vi "ROI_def.vi"(8 "pic path":path, 11 "read image      take pic":bool) -> (0 "Global Rectangle":i32[](array[numeric]), 2 "Image Out 2":T1, 3 "output cluster":cluster{i32, i32, i32, i32})   [LabVIEW 2017]
uses:
  <vilib>/vision/Image Controls.llb/IMAQ Image.ctl
panel:
  in  "Stop (F)":bool
  out "Image Out":T1(plugin-control)
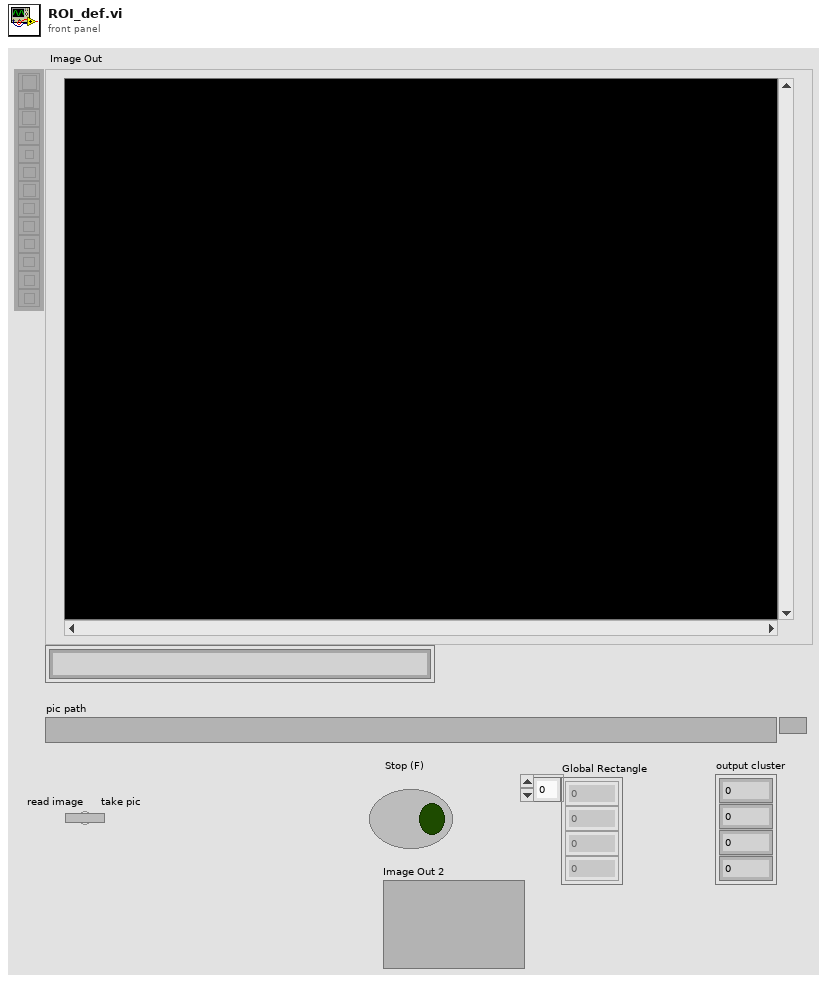
[diagram p1: front panel]
types:
  T1 = typedef "IMAQ Image.ctl" = refnum<image>
  T2 = typedef "ROI Descriptor" = cluster{"Global Rectangle":i32[], "Contours":cluster{"ID":enum32{"External", "Internal"}, "Type":u32, "Coordinates":i32[]}[]}
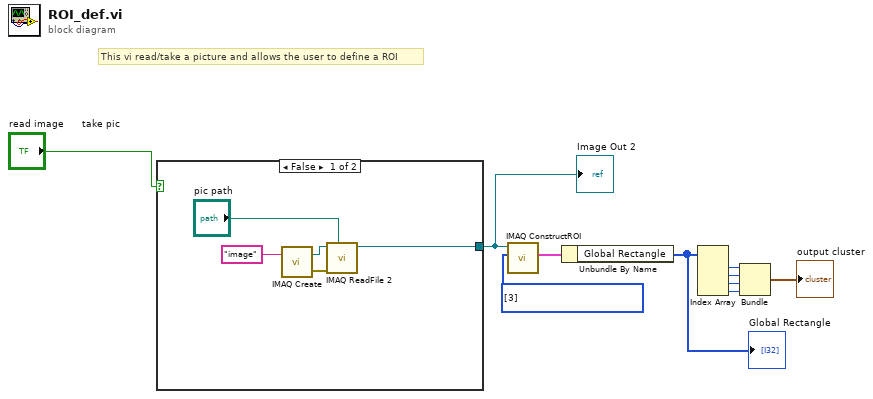
[diagram p0: block diagram]
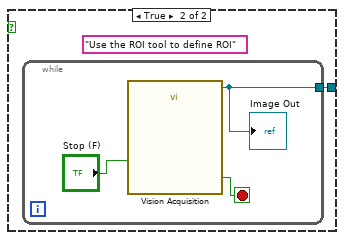
[diagram p2: hidden frame]
diagram:
  w4 = u32[] [3] items=["No Selection", "Point", "Line", "Rectangle", "Oval", "Polygon", "Freehand Region", "Annulus", "Zoom", "Pan", "Broken Line", "Freehand Line", "Rotated Rectangle"] ("Tools")
  # "This vi read/take a picture and allows the user to define a ROI"
  n1 = case shown="False" "read image      take pic" {
    tunnel: [w14 w16] -> w1
    frame False {
      n2 = call "IMAQ Create"("Image Name"="image") -> ("New Image"=w15:T1, "error out"=w12:errorcluster)  [unwired: 4 in]
      n3 = call "IMAQ ReadFile 2"("File Path"="pic path", "error in (no error)"=w12, "Image"=w15) -> ("Image Out"=w14:T1)  [unwired: 4 in, 4 out]
    }
    frame True {
      (unwired) "Use the ROI tool to define ROI" ("Prompt")
      n4 = while {
        tunnel: [w17] -> w16
        stop <- w18 stop-if-true
        n5 = call "Vision Acquisition"("Stop (F)"="Stop (F)") -> ("Image Out"=w17:T1, "Stopped"=w18:bool)  [unwired: 24 in, 1 out]
        "Image Out" <- w17
      }
    }
  }
  "Image Out 2" <- w1
  n6 = call "IMAQ ConstructROI"("Tools"=w4, "Image"=w1) -> ("ROI Descriptor Out"=w10:T2)  [unwired: 6 in, 3 out]
  n7 = Unbundle By Name(w10) -> ("Global Rectangle"=w2:i32[])
  "Global Rectangle" <- w2
  n8 = Index Array(array=w2) -> (element #1=w9:i32, element #2=w8:i32, element #3=w7:i32, element #4=w6:i32)  [unwired: 4 in]
  n9 = Bundle(w9, w8, w7, w6) -> (→"output cluster":cluster{i32, i32, i32, i32})  [unwired: 1 in]
